vi "Save Excluded Devices.vi"(11 "Excluded Devices":string[](array[string])) -> (0 "error IO":errorcluster)   [LabVIEW 2020]
uses:
  <vilib>/Utility/sysdir.llb/System Directory Type.ctl
  <vilib>/Utility/config.llb/NI_LVConfig.lvlib
  <vilib>/Utility/config.llb/Write Key (Boolean).vi
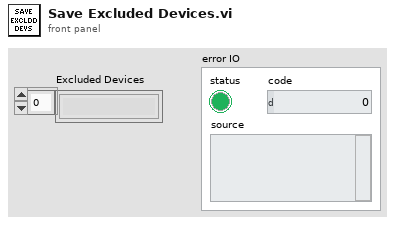
[diagram p1: front panel]
types:
  T1 = typedef "System Directory Type.ctl" = i32
  T2 = typedef "NI_LVConfig.lvlib/Config Data RefNum.ctl" = refnum<k1>
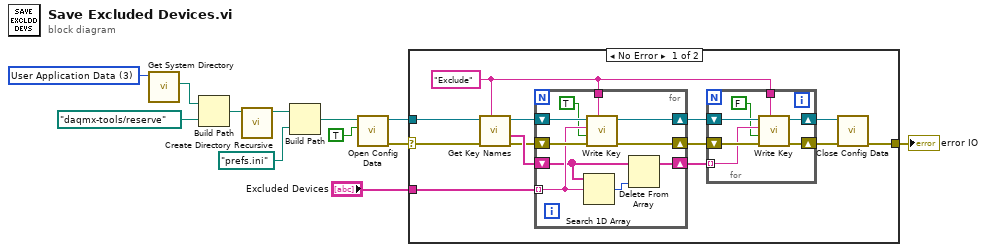
[diagram p0: block diagram]
diagram:
  w12 = T1 3 items=["User Home"=0, "User Desktop"=1, "User Documents"=2, "User Application Data"=3, "User Preferences"=4, "User Temporary"=5, "Public Documents"=6, "Public Application Data"=7, "Public Preferences"=8, "Public Cache"=13, "System Core Libraries"=9, "System Installed Libraries"=10, "Application Files"=11, "Boot Volume Root"=12] ("system directory type")
  n1 = call <vilib>:"Get System Directory.vi"("system directory type"=w12) -> ("system directory"=w11:path)  [unwired: 10 in]
  n2 = Build Path(base path=w11, name or relative path=path "daqmx-tools/reserve") -> (appended path=w9:path)
  n3 = call <vilib>:"Create Directory Recursive.vi"("directory"=w9) -> ("directory copy"=w8:path)  [unwired: 4 in, 2 out]
  n4 = Build Path(base path=w8, name or relative path=path "prefs.ini") -> (appended path=w6:path)
  n5 = call <vilib>:"Open Config Data.vi"("create file if necessary (T)"=TRUE, "configuration file path"=w6) -> ("error out"=w4:errorcluster, "refnum"=w3:T2)  [unwired: 7 in, 1 out]
  n6 = case shown="No Error" w4 {
    selector: w4 -> [w24 w43]
    tunnel: w3 -> [w25 _]
    tunnel: "Excluded Devices" -> [w23 _]
    tunnel: [w13 w43] -> w1
    frame No Error {
      w16 = "Exclude"
      n7 = call <vilib>:"Get Key Names.vi"("section"=w16, "error in (no error)"=w24, "refnum"=w25) -> ("error out"=w20:errorcluster, "key names"=w22:string[], "refnum out"=w21:T2)  [unwired: 5 in, 1 out]
      n8 = for {
        tunnel: w23 -> [w40] mode=indexing
        shift-right: [w36] -> w19
        shift-left: w21 -> [w42]
        shift-right: [w35] -> w18
        shift-left: w20 -> [w41]
        tunnel: w16 -> [w34]
        shift-right: [w37] -> w17
        shift-left: w22 -> [w39]
        n9 = Search 1D Array(1D array=w39, element=w40) -> (index of element=w38:i32)  [unwired: 1 in]
        n10 = call-poly <vilib>:"Write Key.vi"("section"=w34, "error in (no error)"=w41, "value"=TRUE, "key"=w40, "refnum"=w42) -> ("error out"=w35:errorcluster, "refnum out"=w36:T2)  [unwired: 4 in, 1 out]
        n11 = Delete From Array(array=w39, index=w38) -> (array with subset deleted=w37:string[])  [unwired: 1 in, 1 out]
      }
      n12 = for {
        tunnel: w17 -> [w30] mode=indexing
        shift-right: [w29] -> w15
        shift-left: w19 -> [w32]
        shift-right: [w28] -> w14
        shift-left: w18 -> [w31]
        tunnel: w16 -> [w27]
        n13 = call-poly <vilib>:"Write Key.vi"("section"=w27, "error in (no error)"=w31, "value"=FALSE, "key"=w30, "refnum"=w32) -> ("error out"=w28:errorcluster, "refnum out"=w29:T2)  [unwired: 4 in, 1 out]
      }
      n14 = call <vilib>:"Close Config Data.vi"("error in (no error)"=w14, "refnum"=w15) -> ("error out"=w13:errorcluster)  [unwired: 8 in, 1 out]
    }
    frame Error {
    }
  }
  "error IO" <- w1
